vi "Calculate Index Array.vi"(8 "error in (no error)":errorcluster, 10 "3D Ribbon Datatype.lvclass in":refnum<class "3D Ribbon Datatype.lvclass">, 11 "Plot Representation In":T1) -> (0 "error out":errorcluster, 2 "3D Ribbon Datatype.lvclass out":refnum<class "3D Ribbon Datatype.lvclass">, 3 "Plot Representation Out":T1)   [LabVIEW 2017, in "3D Ribbon Datatype.lvclass"]
uses:
  <vilib>/Math Plots/3D Math Plots/3D Ribbon/3D Ribbon Datatype/3D Ribbon Datatype.lvclass
  <vilib>/Math Plots/3D Math Plots/3D Plot/3D Plot/Typedef/Plot Representation.ctl
  <vilib>/Math Plots/3D Math Plots/3D Plot/3D Plot/Typedef/Range Clusters.ctl
  <vilib>/Math Plots/3D Math Plots/3D Plot/3D Plot/Typedef/Mesh Data.ctl
  <vilib>/Math Plots/3D Math Plots/3D Plot/3D Plot/3D Plot.lvclass
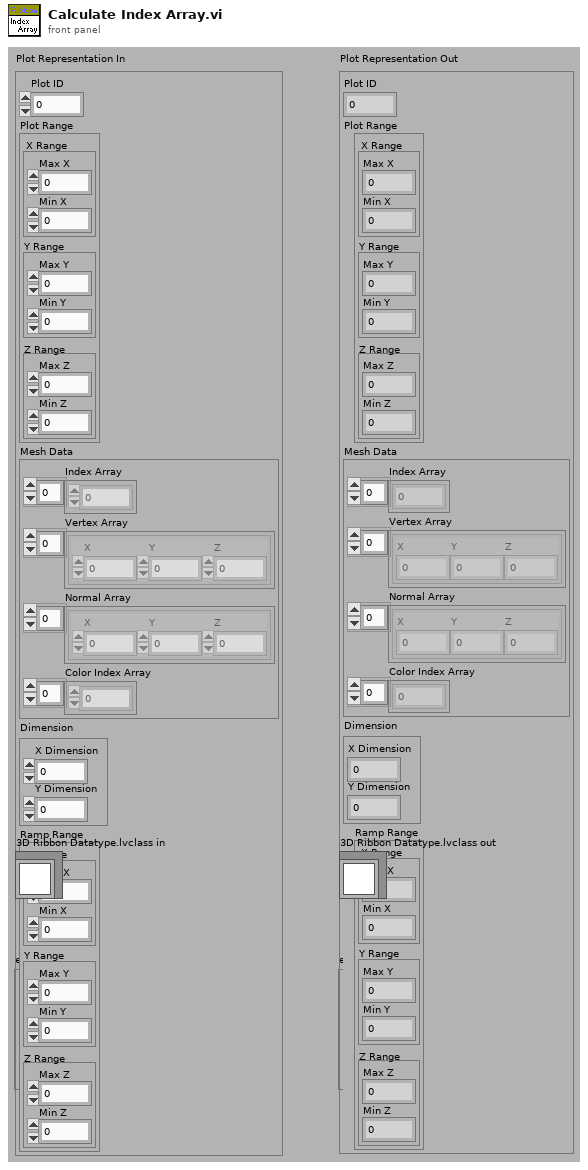
[diagram p1: front panel]
types:
  T1 = typedef "3D Plot.lvclass/Plot Representation.ctl" = cluster{"Plot ID":i32, "Plot Range":T2, "Mesh Data":T3, "Dimension":cluster{"X Dimension":i32, "Y Dimension":i32}, "Ramp Range":T2}
  T2 = typedef "3D Plot.lvclass/Range Clusters.ctl" = cluster{"X Range":cluster{"Max X":sgl, "Min X":sgl}, "Y Range":cluster{"Max Y":sgl, "Min Y":sgl}, "Z Range":cluster{"Max Z":sgl, "Min Z":sgl}}
  T3 = typedef "3D Plot.lvclass/Mesh Data.ctl" = cluster{"Index Array":u32[], "Vertex Array":cluster{"X":sgl, "Y":sgl, "Z":sgl}[], "Normal Array":cluster{"X":sgl, "Y":sgl, "Z":sgl}[], "Color Index Array":i32[]}
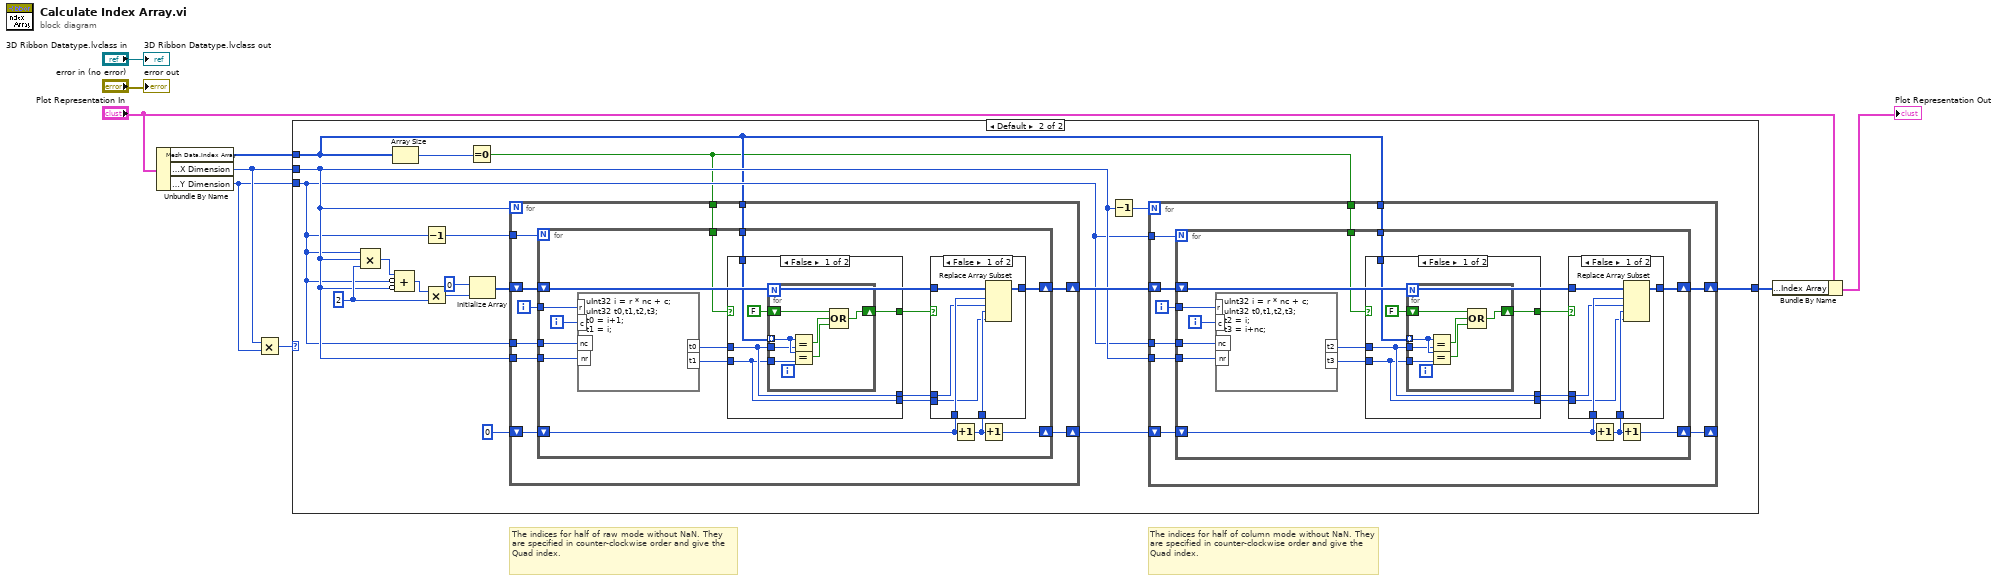
[diagram p0: block diagram]
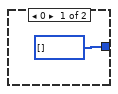
[diagram p2: hidden frame]
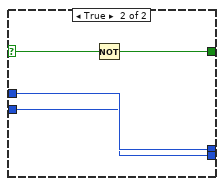
[diagram p4: hidden frame]
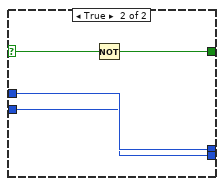
[diagram p6: hidden frame]
diagram:
  # "The indices for half of column mode without NaN. They are specified in counter-clockwise order and give the Quad index."
  # "The indices for half of raw mode without NaN. They are specified in counter-clockwise order and give the Quad index."
  n1 = Unbundle By Name("Plot Representation In") -> ("Mesh Data.Index Array"=w1:u32[], "Dimension.X Dimension"=w3:i32, "Dimension.Y Dimension"=w2:i32)
  n2 = Multiply(x=w3, y=w2) -> (x*y=w4:i32)
  n3 = case shown="Default" w4 {
    tunnel: [u32[] [] w22] -> w5
    tunnel: w2 -> [_ w15]
    tunnel: w3 -> [_ w16]
    tunnel: w1 -> [_ w12]
    frame 0 {
    }
    frame Default {
      w20 = 2 ("y")
      n4 = Compound Arithmetic op=MULTIPLY(w15, w16, w20) -> (w19:i32)
      n5 = Array Size(array=w12) -> (size(s)=w13:i32)
      n6 = Compound Arithmetic op=ADD(w19, invert w15, invert w16) -> (w18:i32)
      n7 = Decrement(x=w15) -> (x-1=w17:i32)
      n8 = Multiply(x=w18, y=w20) -> (x*y=w21:i32)
      n9 = Equal To 0?(x=w13) -> (x = 0?=w11:bool)
      n10 = Initialize Array(u32 0, w21) -> (w26:u32[])
      n11 = for {
        N: w16 -> [_]
        shift-right: [w82] -> w23
        shift-left: w26 -> [w86]
        tunnel: w17 -> [w84]
        tunnel: w15 -> [w83]
        tunnel: w16 -> [w81]
        shift-right: [w80] -> w24
        shift-left: 0 -> [w79]
        tunnel: w11 -> [w78]
        tunnel: w12 -> [w77]
        i -> [w85]
        n12 = for {
          N: w84 -> [_]
          tunnel: w85 -> [w102]
          tunnel: w83 -> [w100]
          shift-right: [w97] -> w82
          shift-left: w86 -> [w98]
          tunnel: w81 -> [w99]
          shift-right: [w94] -> w80
          shift-left: w79 -> [w95]
          tunnel: w78 -> [w89]
          tunnel: w77 -> [w88]
          i -> [w101]
          n13 = formula code="uInt32 i = r * nc + c; \nuInt32 t0,t1,t2,t3;\nt0 = i+1; \nt1 = i;"("r"=w102, "nc"=w100, "c"=w101, "nr"=w99) -> ("t0"=w93:u32, "t1"=w92:u32)
          n14 = case shown="False" w89 {
            selector: w89 -> [_ w123]
            tunnel: [w111 w125] -> w90
            tunnel: w93 -> [w111 w125]
            tunnel: [w110 w124] -> w91
            tunnel: w92 -> [w110 w124]
            tunnel: w88 -> [w114 _]
            tunnel: [w112 w122] -> w87
            frame False {
              n15 = for {
                tunnel: w114 -> [w121] mode=indexing
                tunnel: w111 -> [w120]
                tunnel: w110 -> [w115]
                shift-right: [w117] -> w112
                shift-left: FALSE -> [w116]
                n16 = Equal?(x=w121, y=w120) -> (x = y?=w119:bool)
                n17 = Equal?(x=w121, y=w115) -> (x = y?=w118:bool)
                n18 = Compound Arithmetic op=OR(w116, w119, w118) -> (w117:bool)
              }
            }
            frame True {
              n19 = Not(x=w123) -> (.not. x?=w122:bool)
            }
          }
          n20 = Increment(x=w95) -> (x+1=w96:i32)
          n21 = case shown="False" w87 {
            tunnel: w98 -> [w108 w109]
            tunnel: [w107 w109] -> w97
            tunnel: w96 -> [w106 _]
            tunnel: w95 -> [w105 _]
            tunnel: w91 -> [w104 _]
            tunnel: w90 -> [w103 _]
            frame False {
              n22 = Replace Array Subset(array=w108, new element #1=w103, index #1=w105, new element #2=w104, index #2=w106) -> (w107:u32[])
            }
            frame True {
            }
          }
          n23 = Increment(x=w96) -> (x+1=w94:i32)
        }
      }
      n24 = Decrement(x=w16) -> (x-1=w14:i32)
      n25 = for {
        N: w14 -> [_]
        shift-right: [w33] -> w22
        shift-left: w23 -> [w37]
        tunnel: w15 -> [w35]
        tunnel: w15 -> [w34]
        tunnel: w16 -> [w32]
        shift-right: [w31] -> _
        shift-left: w24 -> [w30]
        tunnel: w12 -> [w29]
        tunnel: w11 -> [w28]
        i -> [w36]
        n26 = for {
          N: w35 -> [_]
          tunnel: w36 -> [w53]
          tunnel: w34 -> [w51]
          shift-right: [w48] -> w33
          shift-left: w37 -> [w49]
          tunnel: w32 -> [w50]
          shift-right: [w45] -> w31
          shift-left: w30 -> [w46]
          tunnel: w29 -> [w44]
          tunnel: w28 -> [w43]
          i -> [w52]
          n27 = formula code="uInt32 i = r * nc + c; \nuInt32 t0,t1,t2,t3;\nt2 = i; \nt3 = i+nc;"("r"=w53, "nc"=w51, "c"=w52, "nr"=w50) -> ("t2"=w42:u32, "t3"=w41:u32)
          n28 = case shown="False" w43 {
            selector: w43 -> [_ w74]
            tunnel: [w62 w76] -> w40
            tunnel: w42 -> [w62 w76]
            tunnel: [w61 w75] -> w39
            tunnel: w41 -> [w61 w75]
            tunnel: w44 -> [w65 _]
            tunnel: [w63 w73] -> w38
            frame False {
              n29 = for {
                tunnel: w65 -> [w72] mode=indexing
                tunnel: w62 -> [w71]
                tunnel: w61 -> [w66]
                shift-right: [w68] -> w63
                shift-left: FALSE -> [w67]
                n30 = Equal?(x=w72, y=w71) -> (x = y?=w70:bool)
                n31 = Equal?(x=w72, y=w66) -> (x = y?=w69:bool)
                n32 = Compound Arithmetic op=OR(w67, w70, w69) -> (w68:bool)
              }
            }
            frame True {
              n33 = Not(x=w74) -> (.not. x?=w73:bool)
            }
          }
          n34 = Increment(x=w46) -> (x+1=w47:i32)
          n35 = case shown="False" w38 {
            tunnel: w49 -> [w59 w60]
            tunnel: [w58 w60] -> w48
            tunnel: w47 -> [w57 _]
            tunnel: w46 -> [w56 _]
            tunnel: w40 -> [w55 _]
            tunnel: w39 -> [w54 _]
            frame False {
              n36 = Replace Array Subset(array=w59, new element #1=w55, index #1=w56, new element #2=w54, index #2=w57) -> (w58:u32[])
            }
            frame True {
            }
          }
          n37 = Increment(x=w47) -> (x+1=w45:i32)
        }
      }
    }
  }
  n38 = Bundle By Name(cluster="Plot Representation In", "Mesh Data.Index Array"=w5) -> (→"Plot Representation Out":T1)
  "error out" <- "error in (no error)"
  "3D Ribbon Datatype.lvclass out" <- "3D Ribbon Datatype.lvclass in"
